vi "CapacitiveTouch Example.vi"() -> ()   [LabVIEW 2012, in "Phidget Capacitive Touch.lvlib"]
uses:
  <instrlib>/Phidgets/Phidget Capacitive Touch/Phidget Capacitive Touch.lvlib
  <instrlib>/Phidgets/Phidget Capacitive Touch/Public/CapacitiveTouchStart.vi
  <instrlib>/Phidgets/Phidget Capacitive Touch/Public/CapacitiveTouchClose.vi
  <instrlib>/Phidgets/Phidget Common/Phidget Common.lvlib
panel:
  out "Touch Input Value":dbl
  out "Is Touched":bool
  out "error out":errorcluster
  in  "error in (no error)":errorcluster
  in  "Device Info":T1={"Serial Number"=-1, "Channel"=0, "Port"=0}
  out "Attached?":bool
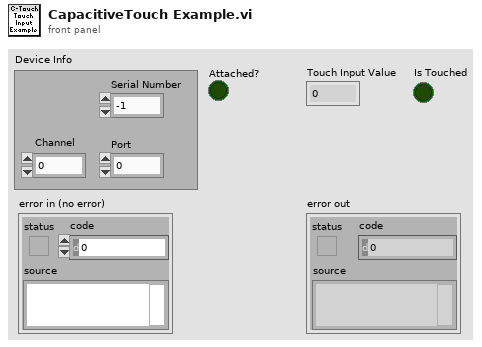
[diagram p1: front panel]
types:
  T1 = cluster{"Serial Number":i32, "Channel":i32, "Port":i32}
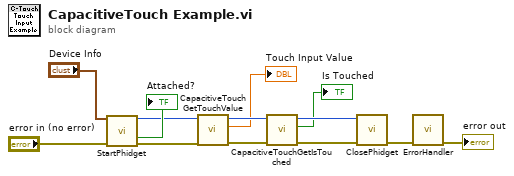
[diagram p0: block diagram]
diagram:
  n1 = call-poly <instrlib>:"StartPhidget.vi"("Device Info"="Device Info", "error in (no error)"="error in (no error)") -> ("Phidget ID"=w8:u64, "Attached?"=→"Attached?":bool, "error out"=w7:errorcluster)  [unwired: 10 in, 1 out]
  n2 = call <instrlib>:"CapacitiveTouchGetTouchValue.vi"("error in (no error)"=w7, "Device In"=w8) -> ("error out"=w5:errorcluster, "Touch Value"=→"Touch Input Value":dbl, "Device Out"=w6:u64)  [unwired: 6 in]
  n3 = call <instrlib>:"CapacitiveTouchGetIsTouched.vi"("error in (no error)"=w5, "Device In"=w6) -> ("error out"=w4:errorcluster, "Is Touched"=→"Is Touched":bool, "Device Out"=w3:u64)  [unwired: 6 in]
  n4 = call-poly <instrlib>:"ClosePhidget.vi"("error in"=w4, "Device In"=w3) -> ("error out"=w10:errorcluster)  [unwired: 9 in]
  n5 = call <instrlib>:"ErrorHandler.vi"("error in"=w10) -> ("error out"=→"error out":errorcluster)  [unwired: 9 in, 1 out]
